vi "checkCmdOrEvent.vi"(8 "error in (no error)":errorcluster, 10 "tcpPacket":T1, 11 "tcpServer in":refnum<class "TcpServer.lvclass">) -> (0 "error out":errorcluster, 2 "typeOfPacket":string, 3 "tcpServer out":refnum<class "TcpServer.lvclass">)   [LabVIEW 2018, in "TcpServer.lvclass"]
doc: "Check if the incoming packet is a command or an event."
uses:
  TcpServer.lvclass
  typedef/tcpPacketTypeDef.ctl
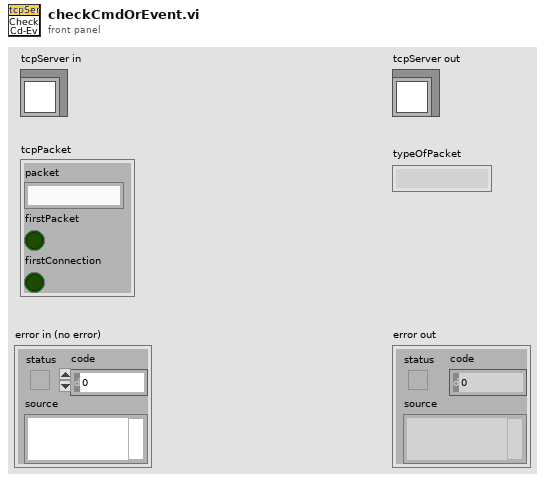
[diagram p1: front panel]
types:
  T1 = typedef "TcpServer.lvclass/tcpPacketTypeDef.ctl" = cluster{"packet":string, "firstPacket":bool, "firstConnection":bool}
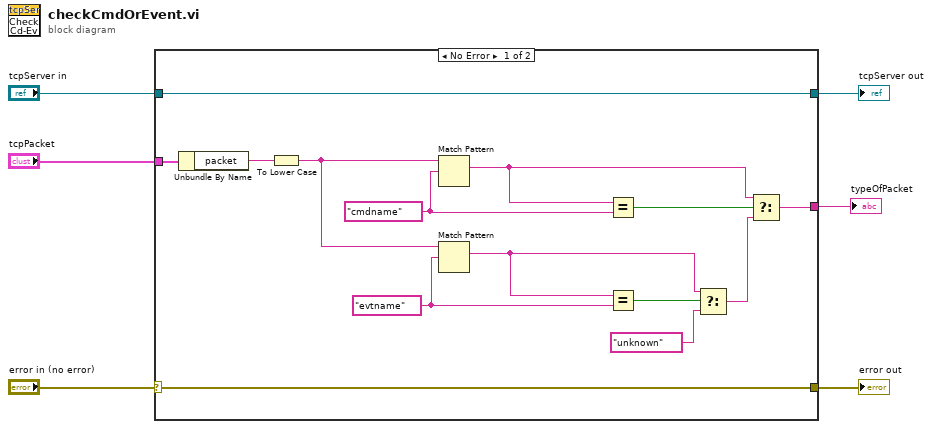
[diagram p0: block diagram]
diagram:
  n1 = case shown="No Error" "error in (no error)" {
    selector: "error in (no error)" -> [w14 w22]
    tunnel: [w14 w22] -> w5
    tunnel: [w20 w21] -> w3
    tunnel: "tcpServer in" -> [w20 w21]
    tunnel: "tcpPacket" -> [w13 _]
    tunnel: [w15 _] -> w1
    frame No Error {
      w7 = "evtname" ("regular expression")
      w8 = "cmdname" ("regular expression")
      n2 = Unbundle By Name(w13) -> ("packet"=w10:string)
      n3 = To Lower Case(string=w10) -> (all lower case string=w9:string)
      n4 = Match Pattern(string=w9, regular expression=w8) -> (match substring=w12:string)  [unwired: 1 in, 3 out]
      n5 = Match Pattern(string=w9, regular expression=w7) -> (match substring=w11:string)  [unwired: 1 in, 3 out]
      n6 = Equal?(x=w12, y=w8) -> (x = y?=w19:bool)
      n7 = Equal?(x=w11, y=w7) -> (x = y?=w18:bool)
      n8 = Select(t=w11, s=w18, f="unknown" ("regular expression")) -> (s? t:f=w17:string)
      n9 = Select(t=w12, s=w19, f=w17) -> (s? t:f=w15:string)
    }
    frame Error {
    }
  }
  "error out" <- w5
  "tcpServer out" <- w3
  "typeOfPacket" <- w1
